vi "IPI_DrawCross.vi"(0 "Image In":T1(plugin-control), 1 "Show Cross":bool=TRUE, 5 "X":dbl, 9 "Y":dbl=150.0, 11 "error in (no error)":errorcluster, 12 "Radius":dbl=150.0, 13 "颜色盒":u32(colorbox)=16711680) -> (4 "Image Out":T1(plugin-control), 15 "error out":errorcluster)   [LabVIEW 2015]
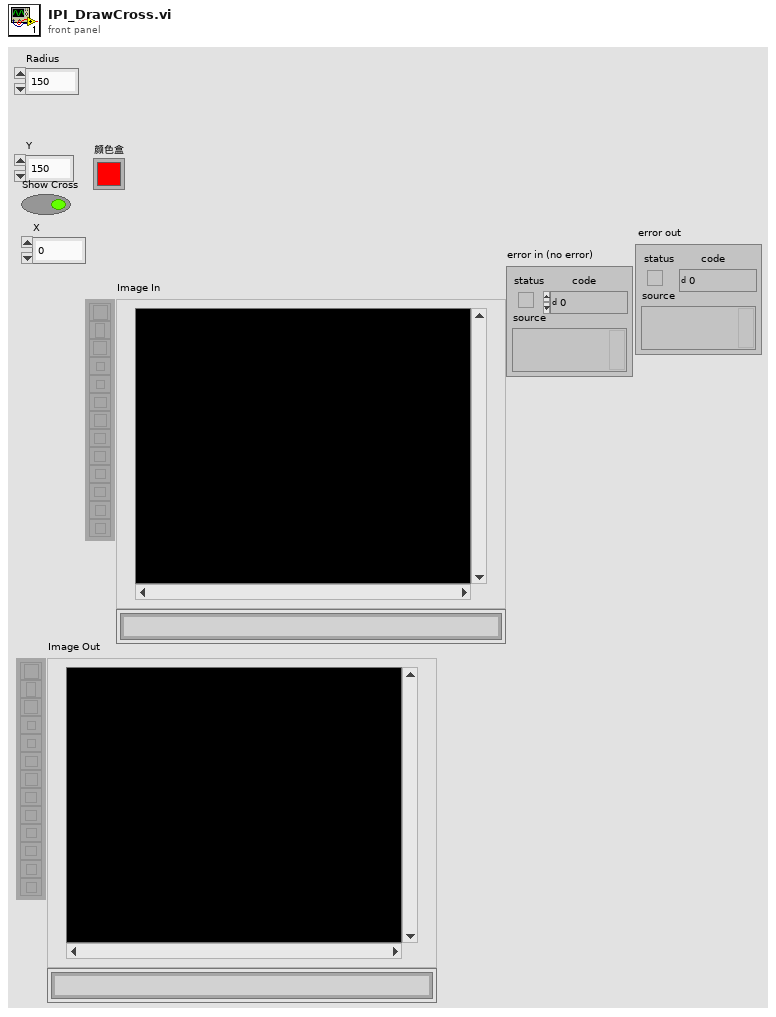
[diagram p1: front panel]
types:
  T1 = typedef "IMAQ Image.ctl" = refnum<image>
  T2 = cluster{"Left":i32, "Top":i32, "Right":i32, "Bottom":i32}
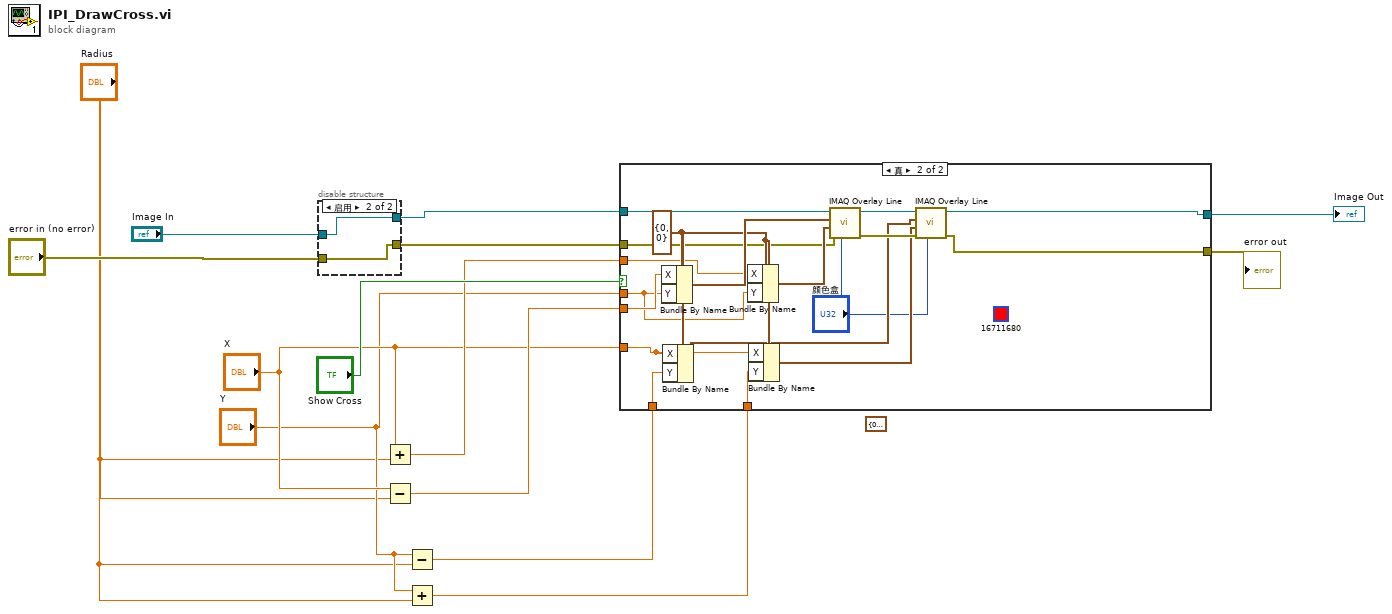
[diagram p0: block diagram]
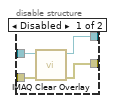
[diagram p2: hidden frame]
diagram:
  (unwired) T2 {"Left"=0, "Top"=0, "Right"=0, "Bottom"=0} ("Bounding Rectangle")
  n1 = disable-structure shown="启用" {
    disable-tunnel: "Image In" -> [w18 w20]
    disable-tunnel: [w17 w20] -> w13
    disable-tunnel: "error in (no error)" -> [w16 w19]
    disable-tunnel: [w15 w19] -> w8
    frame Disabled {
      n2 = call "IMAQ Clear Overlay"("error in (no error)"=w16, "Image"=w18) -> ("error out"=w15:errorcluster, "Image Out"=w17:T1)  [unwired: 8 in]
    }
    frame Enabled {
    }
  }
  n3 = Add(x="X", y="Radius") -> (x+y=w6:dbl)
  n4 = Subtract(x="X", y="Radius") -> (x-y=w7:dbl)
  n5 = Subtract(x="Y", y="Radius") -> (x-y=w2:dbl)
  n6 = Add(x="Y", y="Radius") -> (x+y=w1:dbl)
  n7 = case shown="真" "Show Cross" {
    tunnel: w13 -> [w22 w40]
    tunnel: [w22 w30] -> w12
    tunnel: [w21 w29] -> w10
    tunnel: w8 -> [w21 w31]
    tunnel: "Y" -> [_ w27]
    tunnel: w7 -> [_ w28]
    tunnel: w6 -> [_ w26]
    tunnel: "X" -> [_ w25]
    tunnel: w2 -> [_ w24]
    tunnel: w1 -> [_ w23]
    frame False {
    }
    frame True {
      (unwired) u32 16711680
      w35 = cluster{"X":i32, "Y":i32} {"X"=0, "Y"=0} ("Start Point")
      n8 = Bundle By Name(cluster=w35, "X"=w28, "Y"=w27) -> (w39:cluster{"X":i32, "Y":i32})
      n9 = Bundle By Name(cluster=w35, "X"=w25, "Y"=w24) -> (w33:cluster{"X":i32, "Y":i32})
      n10 = Bundle By Name(cluster=w35, "X"=w26, "Y"=w27) -> (w38:cluster{"X":i32, "Y":i32})
      n11 = Bundle By Name(cluster=w35, "X"=w25, "Y"=w23) -> (w34:cluster{"X":i32, "Y":i32})
      n12 = call "IMAQ Overlay Line"("Color"="颜色盒", "error in (no error)"=w31, "End Point"=w38, "Start Point"=w39, "Image"=w40) -> ("error out"=w36:errorcluster, "Image Out"=w37:T1)  [unwired: 5 in]
      n13 = call "IMAQ Overlay Line"("Color"="颜色盒", "error in (no error)"=w36, "End Point"=w34, "Start Point"=w33, "Image"=w37) -> ("error out"=w29:errorcluster, "Image Out"=w30:T1)  [unwired: 5 in]
    }
  }
  "Image Out" <- w12
  "error out" <- w10
